vi "查询上序合格.vi"(8 "error in (no error)":errorcluster, 11 "产品ID":string="123456") -> (0 "error out":errorcluster, 1 "本序已做":bool, 2 "上序合格":bool)   [LabVIEW 2013]
uses:
  <vilib>/Utility/error.llb/whitespace.ctl
panel:
  out "EOF":bool
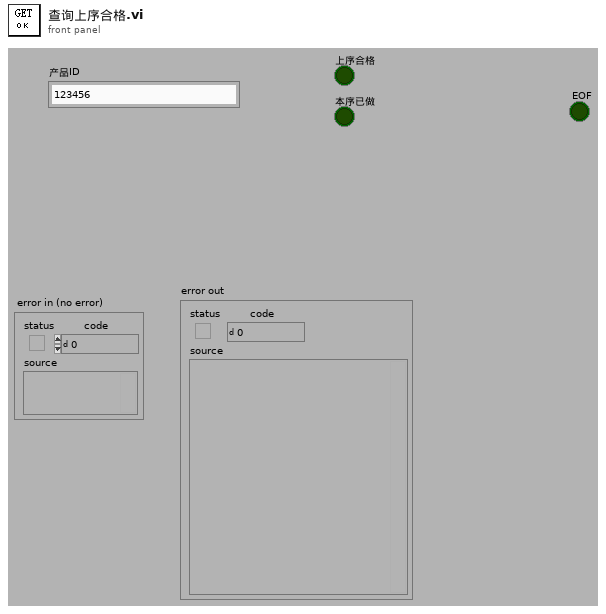
[diagram p1: front panel]
types:
  T1 = typedef "whitespace.ctl" = u16
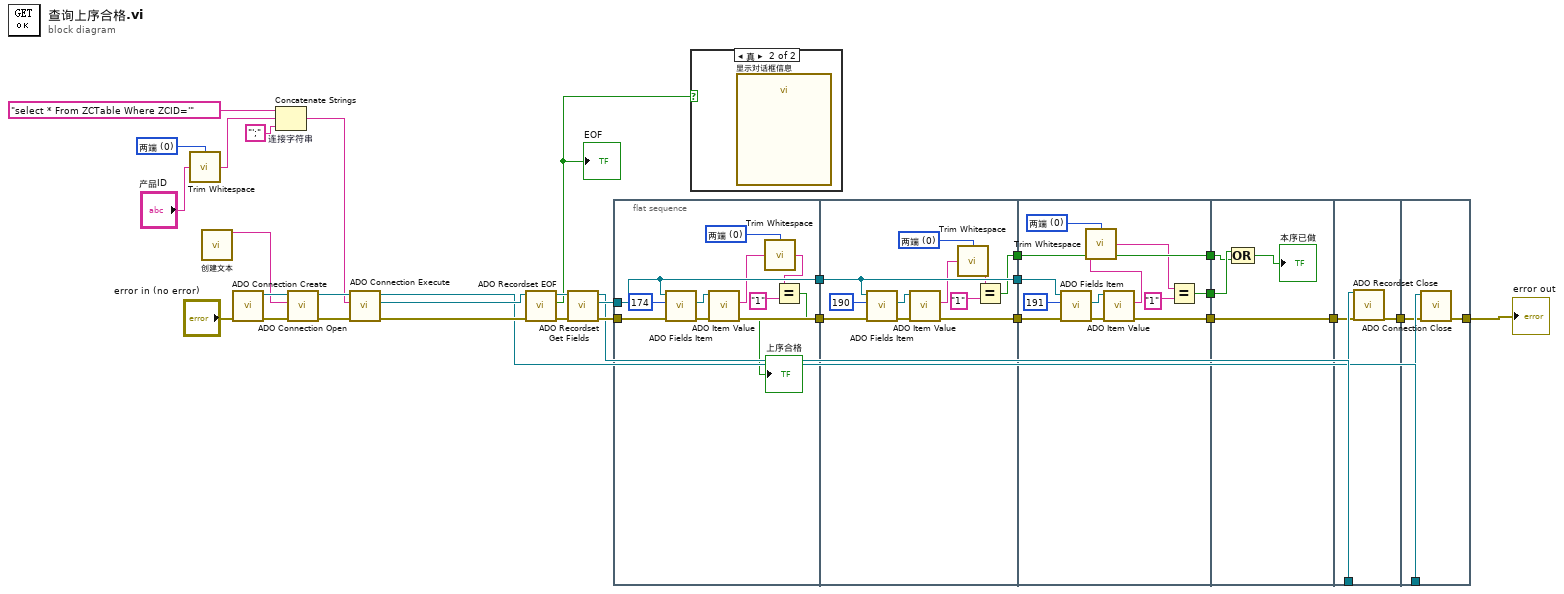
[diagram p0: block diagram]
diagram:
  w22 = T1 0 items=["两端", "字符串首端", "字符串末端"] ("location (both)")
  n1 = call <vilib>:"Trim Whitespace.vi"("string"="产品ID", "location (both)"=w22) -> ("trimmed string"=w23:string)
  n2 = call "创建文本"() -> ("Result"=w2:string)  [unwired: 14 in, 1 out]
  n3 = call "ADO Connection Create.vi"("error in (no error)"="error in (no error)") -> ("error out"=w31:errorcluster, "ADODB._Connection Out"=w32:refnum<k7>)  [unwired: 9 out]
  n4 = Concatenate Strings "连接字符串"("select * From ZCTable Where ZCID='" ("字符串 2"), w23, "';" ("字符串 2")) -> (w21:string)
  n5 = call "ADO Connection Open.vi"("error in (no error)"=w31, "ConnectionString"=w2, "ADODB._Connection In"=w32) -> ("error out"=w30:errorcluster, "ADODB._Connection Out"=w29:refnum<k7>)  [unwired: 7 out]
  n6 = call "ADO Connection Execute.vi"("error in (no error)"=w30, "CommandText"=w21, "ADODB._Connection In"=w29) -> ("error out"=w27:errorcluster, "RecordSet"=w28:refnum<k7>, "ADODB._Connection Out"=w13:refnum<k7>)  [unwired: 6 out]
  n7 = call "ADO Recordset EOF.vi"("error in (no error)"=w27, "ADODB._Recordset In"=w28) -> ("error out"=w18:errorcluster, "EOF"=w1:bool, "ADODB._Recordset Out"=w19:refnum<k7>)  [unwired: 7 out]
  "EOF" <- w1
  n8 = call "ADO Recordset Get Fields.vi"("error in (no error)"=w18, "ADODB._Recordset In"=w19) -> ("error out"=w16:errorcluster, "Fields Out"=w17:refnum<k7>, "ADODB._Recordset Out"=w14:refnum<k7>)  [unwired: 7 out]
  n9 = flat-sequence {
    tunnel: w17 -> [w38]
    tunnel: w16 -> [w39]
    tunnel: [w43] -> w10
    tunnel: [w38] -> w9
    tunnel: w10 -> [w51]
    tunnel: w9 -> [w48]
    tunnel: [w50] -> w7
    tunnel: [w48] -> w6
    tunnel: [w47] -> w4
    tunnel: [w62] -> w8
    tunnel: w7 -> [w63]
    tunnel: w6 -> [w60]
    tunnel: [w59] -> w5
    tunnel: w4 -> [w58]
    tunnel: [w58] -> w3
    tunnel: w8 -> [w70]
    tunnel: [w70] -> w15
    tunnel: w5 -> [w69]
    tunnel: w3 -> [w68]
    tunnel: w15 -> [w72]
    tunnel: w14 -> [w73]
    tunnel: [w71] -> w12
    tunnel: w13 -> [w76]
    tunnel: w12 -> [w75]
    tunnel: [w74] -> w11
    frame #0 {
      w36 = T1 0 items=["两端", "字符串首端", "字符串末端"] ("location (both)")
      n10 = call "ADO Fields Item.vi"("error in (no error)"=w39, "Index"=174, "Fields In"=w38) -> ("error out"=w41:errorcluster, "Item Out"=w40:refnum<k7>)  [unwired: 7 out]
      n11 = call "ADO Item Value.vi"("error in (no error)"=w41, "Item In"=w40) -> ("error out"=w43:errorcluster, "Value"=w35:string)  [unwired: 8 out]
      n12 = call <vilib>:"Trim Whitespace.vi"("string"=w35, "location (both)"=w36) -> ("trimmed string"=w34:string)
      n13 = Equal?(x=w34, y="1") -> (x = y?=→"上序合格":bool)
    }
    frame #1 {
      w46 = T1 0 items=["两端", "字符串首端", "字符串末端"] ("location (both)")
      n14 = call "ADO Fields Item.vi"("error in (no error)"=w51, "Index"=190, "Fields In"=w48) -> ("error out"=w53:errorcluster, "Item Out"=w52:refnum<k7>)  [unwired: 7 out]
      n15 = call "ADO Item Value.vi"("error in (no error)"=w53, "Item In"=w52) -> ("error out"=w50:errorcluster, "Value"=w45:string)  [unwired: 8 out]
      n16 = call <vilib>:"Trim Whitespace.vi"("string"=w45, "location (both)"=w46) -> ("trimmed string"=w44:string)
      n17 = Equal?(x=w44, y="1") -> (x = y?=w47:bool)
    }
    frame #2 {
      w57 = T1 0 items=["两端", "字符串首端", "字符串末端"] ("location (both)")
      n18 = call "ADO Fields Item.vi"("error in (no error)"=w63, "Index"=191, "Fields In"=w60) -> ("error out"=w65:errorcluster, "Item Out"=w64:refnum<k7>)  [unwired: 7 out]
      n19 = call "ADO Item Value.vi"("error in (no error)"=w65, "Item In"=w64) -> ("error out"=w62:errorcluster, "Value"=w56:string)  [unwired: 8 out]
      n20 = call <vilib>:"Trim Whitespace.vi"("string"=w56, "location (both)"=w57) -> ("trimmed string"=w55:string)
      n21 = Equal?(x=w55, y="1") -> (x = y?=w59:bool)
    }
    frame #3 {
      n22 = Compound Arithmetic op=OR(w69, w68) -> (→"本序已做":bool)
    }
    frame #4 {
      n23 = call "ADO Recordset Close.vi"("ADODB._Recordset In"=w73, "error in (no error)"=w72) -> ("error out"=w71:errorcluster)  [unwired: 17 out]
    }
    frame #5 {
      n24 = call "ADO Connection Close.vi"("error in (no error)"=w75, "ADODB._Connection In"=w76) -> ("error out"=w74:errorcluster)  [unwired: 9 out]
    }
  }
  n25 = case shown="真" w1 {
    frame False {
    }
    frame True {
      n26 = call "显示对话框信息"() -> ()  [unwired: 10 in, 2 out]
    }
  }
  "error out" <- w11
